vi "configureSerial.vi"(8 "error in (no error)":errorcluster, 10 "SerialConfig":T1={"VISA resource name"="", "Baud Rate"=9600, "Data Bits"=8, "Parity"=enum."None", "Stop Bits"=10, "Flow Control"=0, "Timeout (ms)"=10000, "Serial Protocol"=enum."RS485"} {"Stop Bits" items=["1.0"=10, "1.5"=15, "2.0"=20]; "Flow Control" items=["None", "XON/XOFF", "RTS/CTS", "XON/XOFF & RTS/CTS", "DTR/DSR", "XON/XOFF & DTR/DSR"]; "Data Bits" min=5 max=8 step=1}, 11 "Model in":refnum<class "Model.lvclass">) -> (0 "error out":errorcluster, 3 "Model out":refnum<class "Model.lvclass">)   [LabVIEW 2013, in "Model.lvclass"]
uses:
  Model.lvclass
  <userlib>/Common/SerialProtocols/Configuration/SerialConfig.ctl
  <userlib>/Common/SerialProtocols/Configuration/SerialProtocol.ctl
  Model.lvclass/Model.ctl
  <userlib>/Common/SerialProtocols/SerialCommFactory/ISerialCommFactory/ISerialCommFactory.lvclass
  <userlib>/Common/SerialProtocols/SerialCommunicator/SerialCommunicator/SerialCommunicator.lvclass
  <userlib>/Common/SerialProtocols/SerialProtocols.lvlib
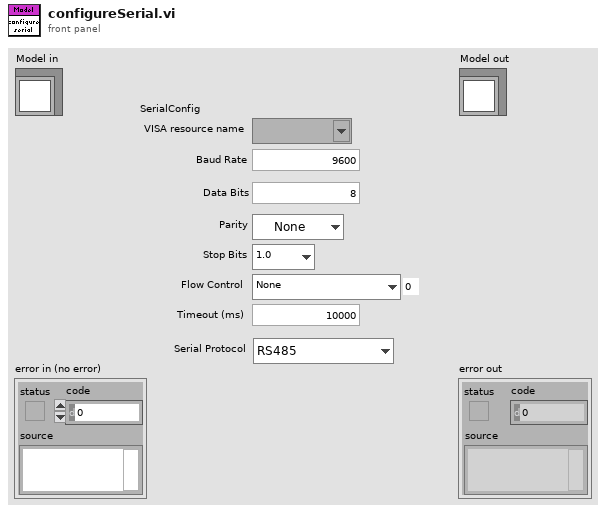
[diagram p1: front panel]
types:
  T1 = typedef "SerialProtocols.lvlib/SerialConfig.ctl" = cluster{"VISA resource name":refnum<visa-resource-name>, "Baud Rate":u32, "Data Bits":u16, "Parity":enum16{"None", "Odd", "Even", "Mark", "Space"}, "Stop Bits":u16, "Flow Control":u16, "Timeout (ms)":u32, "Serial Protocol":T2}
  T2 = typedef "SerialProtocols.lvlib/SerialProtocol.ctl" = enum16{"RS232", "RS485", "SerialSimulator"}
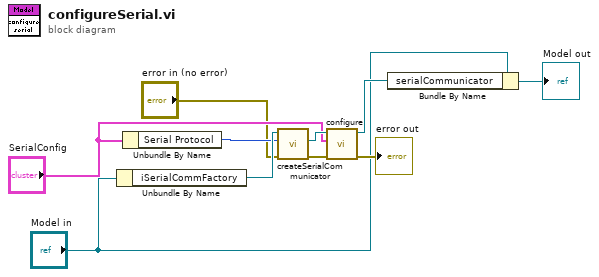
[diagram p0: block diagram]
diagram:
  n1 = Unbundle By Name("Model in") -> ("iSerialCommFactory"=w6:refnum<class "ISerialCommFactory.lvclass">)
  n2 = Unbundle By Name("SerialConfig") -> ("Serial Protocol"=w3:T2)
  n3 = call-dynamic "createSerialCommunicator.vi"("error in (no error)"="error in (no error)", "Serial Protocol"=w3, "ISerialCommFactory in"=w6) -> ("error out"=w1:errorcluster, "serialCommunicator"=w5:refnum<class "SerialCommunicator.lvclass">)  [unwired: 6 in, 1 out]
  n4 = call-dynamic "configure.vi"("error in (no error)"=w1, "SerialConfig"="SerialConfig", "SerialCommunicator in"=w5) -> ("error out"=→"error out":errorcluster, "SerialCommunicator out"=w8:refnum<class "SerialCommunicator.lvclass">)  [unwired: 7 in]
  n5 = Bundle By Name(cluster="Model in", "serialCommunicator"=w8) -> (→"Model out":refnum<class "Model.lvclass">)
